vi "Get Count Convert Wavelength Range.vi"(10 "maxval":sgl, 11 "minval":sgl) -> (1 "function return":u32, 2 "maxval out":sgl, 3 "minval out":sgl)   [LabVIEW 2018, in "AndorSDK.lvlib"]
doc: "EXPNETTYPE unsigned int WINAPI GetCountConvertWavelengthRange(float * minval, float * maxval);"
uses:
  AndorSDK.lvlib
  ATMCD32D.dll
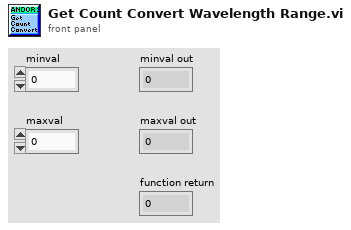
[diagram p1: front panel]
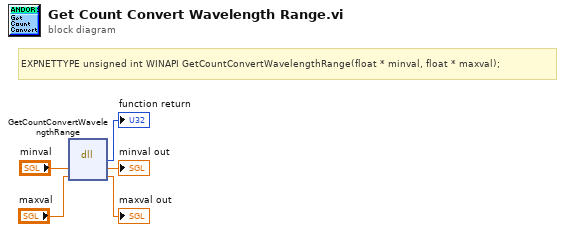
[diagram p0: block diagram]
diagram:
  # "EXPNETTYPE unsigned int WINAPI GetCountConvertWavelengthRange(float * minval, float * maxval);"
  n1 = dll-call lib="PTH2babs E\nPersönliches02 - Arbeit03-HiwijobsLabviewCodelibANDOR\tAndor SDK\nATMCD32D.*" fn="GetCountConvertWavelengthRange"("minval"="minval", "maxval"="maxval") -> (→"function return":u32, "minval"=→"minval out":sgl, "maxval"=→"maxval out":sgl)  [unwired: 3 in, 2 out]
